vi "getDigitalIn.vi"(7 "Device":i32, 8 "error in (no error)":errorcluster, 9 "DigIn":u8, 10 "DigInId":u8, 11 "SEDSpectrometer in":refnum<class "SEDSpectrometer.lvclass">) -> (0 "error out":errorcluster, 1 "DigIn":u8, 2 "Output Value":i32, 3 "SEDSpectrometer out":refnum<class "SEDSpectrometer.lvclass">)   [LabVIEW 2016, in "SEDSpectrometer.lvclass"]
uses:
  SEDSpectrometer.lvclass
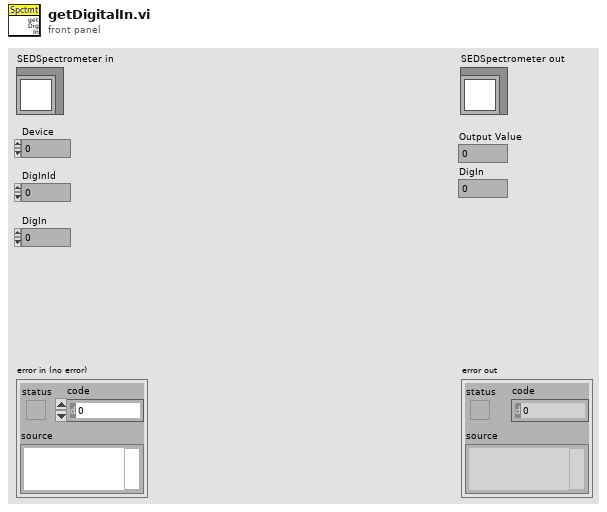
[diagram p1: front panel]
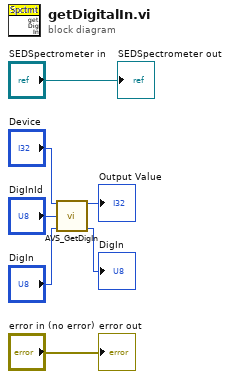
[diagram p0: block diagram]
diagram:
  n1 = call "AVS_GetDigIn.vi"("a_hDevice"="Device", "a_DigInId"="DigInId", "a_pDigIn"="DigIn") -> ("Output Value"=→"Output Value":i32, "a_pDigIn"=→"DigIn":u8)  [unwired: 11 in]
  "error out" <- "error in (no error)"
  "SEDSpectrometer out" <- "SEDSpectrometer in"
